vi "RemoteControlClient.vi"(8 "error in (no error)":errorcluster, 9 "servicePort (9002)":i32=9002, 10 "(localhost)":string="127.0.0.1") -> (0 "error out":errorcluster, 3 "VGS_RemoteControlClient out":refnum<class "VGS_RemoteControlClient.lvclass">)   [LabVIEW 2022 SP3, in "LV_VGS.lvlib" / "VGS_RemoteControlClient.lvclass"]
doc: "Constructs a new instance of RemoteControlClient class."
uses:
  VGS_RemoteControlClient.lvclass
  VGS_RemoteControlClient.lvclass/VGS_RemoteControlClient.ctl
  C:/Users/Andrey/Desktop/hajo/LV_VGS/vgs_project.dll
  vgs_project.dll
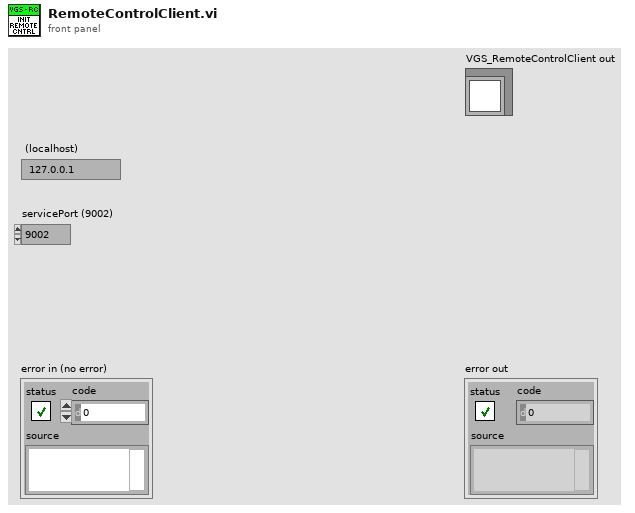
[diagram p1: front panel]
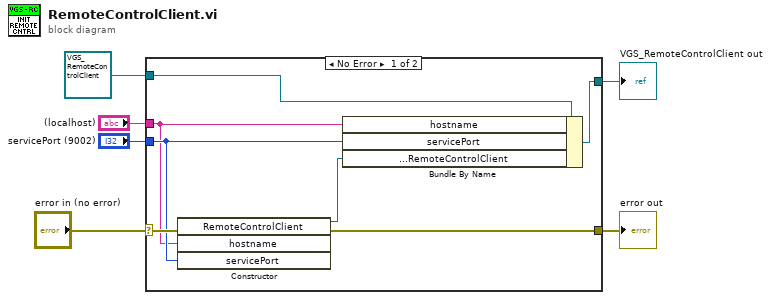
[diagram p0: block diagram]
diagram:
  n1 = case shown="No Error" "error in (no error)" {
    selector: "error in (no error)" -> [w12 w15]
    tunnel: [w11 w15] -> w5
    tunnel: [w13 w14] -> w4
    tunnel: "(localhost)" -> [w9 _]
    tunnel: "servicePort (9002)" -> [w10 _]
    tunnel: refnum<class "VGS_RemoteControlClient.lvclass"> refnum ("VGS_RemoteControlClient in") -> [w7 w14]
    frame No Error {
      n2 = constructor class="RemoteControlClient"(error in=w12, "hostname"=w9, "servicePort"=w10) -> (reference out=w8:refnum<k24>, error out=w11:errorcluster)  [unwired: 2 in, 3 out]
      n3 = Bundle By Name(cluster=w7, "hostname"=w9, "servicePort"=w10, "VGS.Project.Interop.RemoteControlClient"=w8) -> (w13:refnum<class "VGS_RemoteControlClient.lvclass">)
    }
    frame Error {
    }
  }
  "error out" <- w5
  "VGS_RemoteControlClient out" <- w4
